vi "Create Default Font.vi"() -> (3 "Theme.Font out":refnum<class "Theme.Font.lvclass">)   [LabVIEW 2017, in "Theme.lvlib" / "Theme.Font.lvclass"]
uses:
  Theme.Font.lvclass
  Theme.Font.lvclass/Theme.Font.ctl
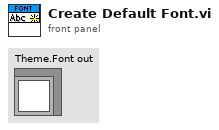
[diagram p1: front panel]
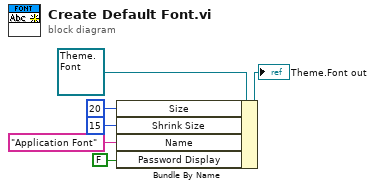
[diagram p0: block diagram]
diagram:
  n1 = Bundle By Name(cluster=refnum<class "Theme.Font.lvclass"> refnum ("Theme.Font in"), "Size"=u32 20, "Shrink Size"=u32 15, "Name"="Application Font", "Password Display"=FALSE ("Font.Password Display")) -> (→"Theme.Font out":refnum<class "Theme.Font.lvclass">)
